vi "TSCANfd_Table.vi"(10 "y":T1(array[cluster]), 11 "MCListbox引用句柄":refnum<vi>) -> ()   [LabVIEW 2019]
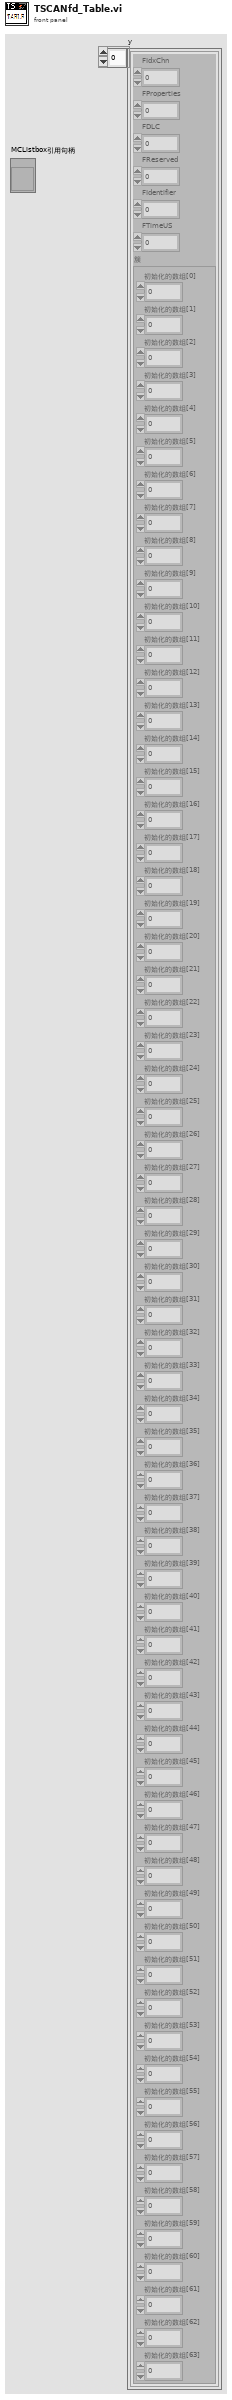
[diagram p1: front panel]
types:
  T1 = cluster{"FIdxChn":u8, "FProperties":u8, "FDLC":u8, "FReserved":u8, "FIdentifier":i32, "FTimeUS":u64, "簇":cluster{"初始化的数组[0]":u8, "初始化的数组[1]":u8, "初始化的数组[2]":u8, "初始化的数组[3]":u8, "初始化的数组[4]":u8, "初始化的数组[5]":u8, "初始化的数组[6]":u8, "初始化的数组[7]":u8, "初始化的数组[8]":u8, "初始化的数组[9]":u8, "初始化的数组[10]":u8, "初始化的数组[11]":u8, "初始化的数组[12]":u8, "初始化的数组[13]":u8, "初始化的数组[14]":u8, "初始化的数组[15]":u8, "初始化的数组[16]":u8, "初始化的数组[17]":u8, "初始化的数组[18]":u8, "初始化的数组[19]":u8, "初始化的数组[20]":u8, "初始化的数组[21]":u8, "初始化的数组[22]":u8, "初始化的数组[23]":u8, "初始化的数组[24]":u8, "初始化的数组[25]":u8, "初始化的数组[26]":u8, "初始化的数组[27]":u8, "初始化的数组[28]":u8, "初始化的数组[29]":u8, "初始化的数组[30]":u8, "初始化的数组[31]":u8, "初始化的数组[32]":u8, "初始化的数组[33]":u8, "初始化的数组[34]":u8, "初始化的数组[35]":u8, "初始化的数组[36]":u8, "初始化的数组[37]":u8, "初始化的数组[38]":u8, "初始化的数组[39]":u8, "初始化的数组[40]":u8, "初始化的数组[41]":u8, "初始化的数组[42]":u8, "初始化的数组[43]":u8, "初始化的数组[44]":u8, "初始化的数组[45]":u8, "初始化的数组[46]":u8, "初始化的数组[47]":u8, "初始化的数组[48]":u8, "初始化的数组[49]":u8, "初始化的数组[50]":u8, "初始化的数组[51]":u8, "初始化的数组[52]":u8, "初始化的数组[53]":u8, "初始化的数组[54]":u8, "初始化的数组[55]":u8, "初始化的数组[56]":u8, "初始化的数组[57]":u8, "初始化的数组[58]":u8, "初始化的数组[59]":u8, "初始化的数组[60]":u8, "初始化的数组[61]":u8, "初始化的数组[62]":u8, "初始化的数组[63]":u8}}[]
  T2 = cluster{"初始化的数组[0]":u8, "初始化的数组[1]":u8, "初始化的数组[2]":u8, "初始化的数组[3]":u8, "初始化的数组[4]":u8, "初始化的数组[5]":u8, "初始化的数组[6]":u8, "初始化的数组[7]":u8, "初始化的数组[8]":u8, "初始化的数组[9]":u8, "初始化的数组[10]":u8, "初始化的数组[11]":u8, "初始化的数组[12]":u8, "初始化的数组[13]":u8, "初始化的数组[14]":u8, "初始化的数组[15]":u8, "初始化的数组[16]":u8, "初始化的数组[17]":u8, "初始化的数组[18]":u8, "初始化的数组[19]":u8, "初始化的数组[20]":u8, "初始化的数组[21]":u8, "初始化的数组[22]":u8, "初始化的数组[23]":u8, "初始化的数组[24]":u8, "初始化的数组[25]":u8, "初始化的数组[26]":u8, "初始化的数组[27]":u8, "初始化的数组[28]":u8, "初始化的数组[29]":u8, "初始化的数组[30]":u8, "初始化的数组[31]":u8, "初始化的数组[32]":u8, "初始化的数组[33]":u8, "初始化的数组[34]":u8, "初始化的数组[35]":u8, "初始化的数组[36]":u8, "初始化的数组[37]":u8, "初始化的数组[38]":u8, "初始化的数组[39]":u8, "初始化的数组[40]":u8, "初始化的数组[41]":u8, "初始化的数组[42]":u8, "初始化的数组[43]":u8, "初始化的数组[44]":u8, "初始化的数组[45]":u8, "初始化的数组[46]":u8, "初始化的数组[47]":u8, "初始化的数组[48]":u8, "初始化的数组[49]":u8, "初始化的数组[50]":u8, "初始化的数组[51]":u8, "初始化的数组[52]":u8, "初始化的数组[53]":u8, "初始化的数组[54]":u8, "初始化的数组[55]":u8, "初始化的数组[56]":u8, "初始化的数组[57]":u8, "初始化的数组[58]":u8, "初始化的数组[59]":u8, "初始化的数组[60]":u8, "初始化的数组[61]":u8, "初始化的数组[62]":u8, "初始化的数组[63]":u8}
  T3 = typedef "LVRowAndColumnUnsignedTypeDef.ctl" = cluster{"Row":u32, "Column":u32}
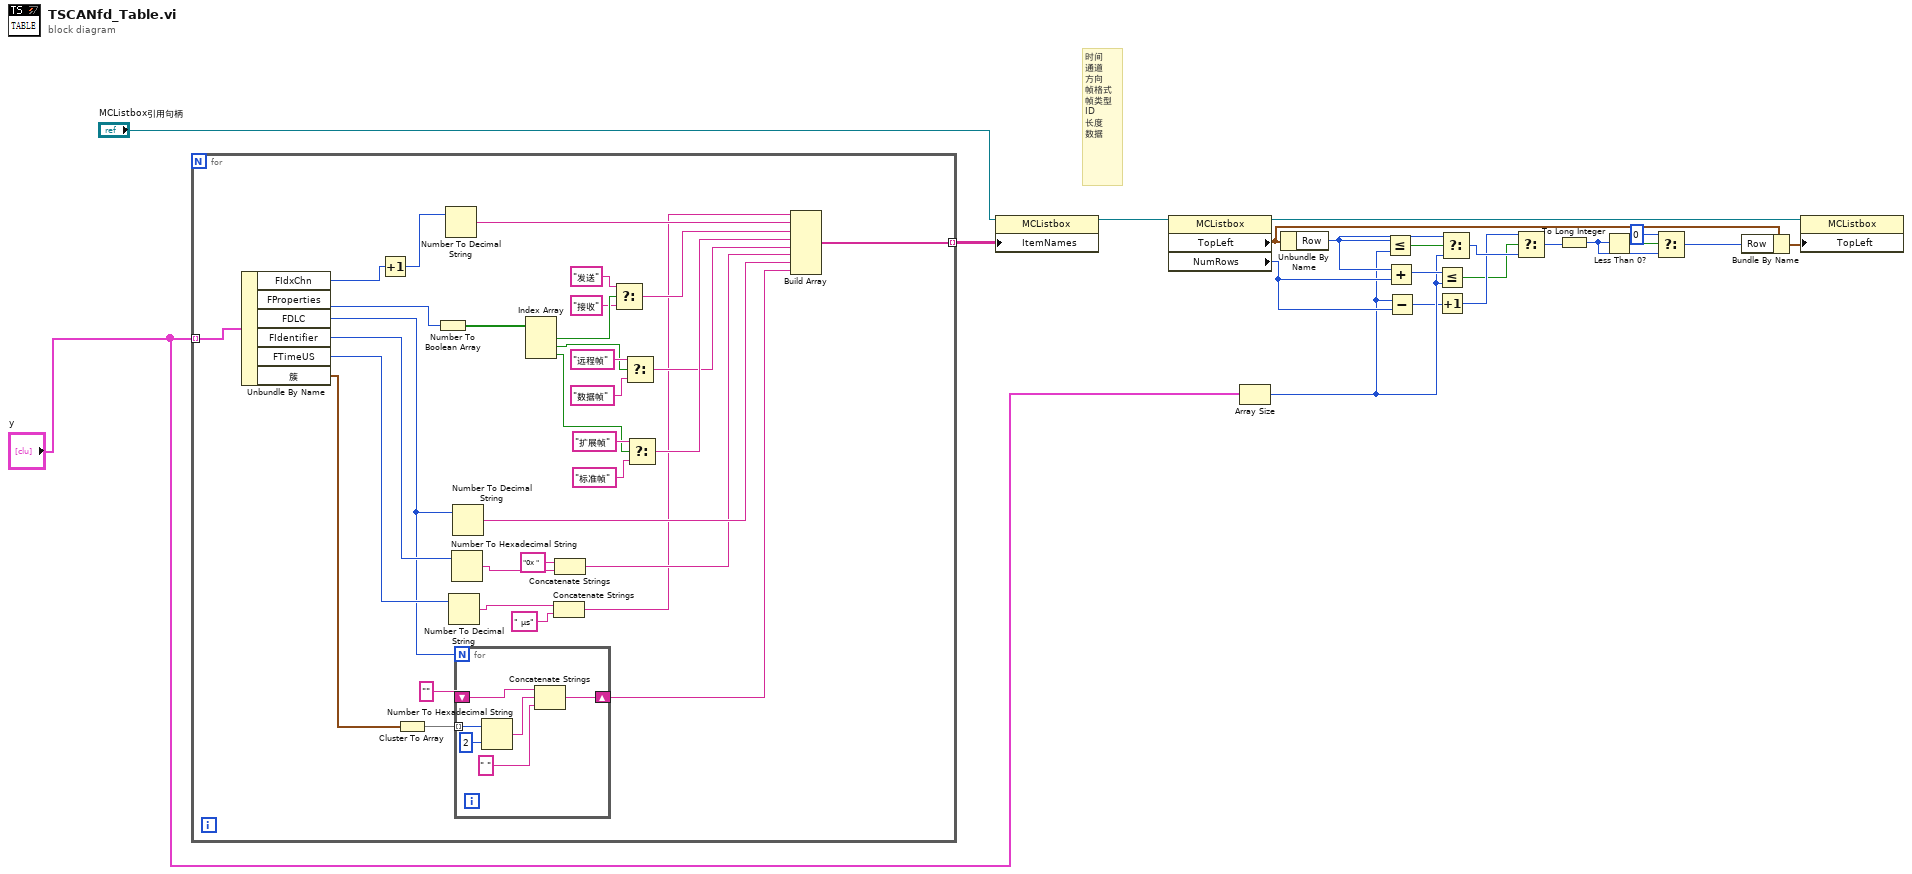
[diagram p0: block diagram]
diagram:
  # "时间\n通道\n方向\n帧格式\n帧类型\nID\n长度\n数据"
  n1 = for {
    tunnel: "y" -> [w54] mode=indexing
    tunnel: [w30] -> w21 mode=indexing
    n2 = Unbundle By Name(w54) -> ("FIdxChn"=w29:u8, "FProperties"=w53:u8, "FDLC"=w38:u8, "FIdentifier"=w42:i32, "FTimeUS"=w41:u64, "簇"=w39:T2)
    n3 = Increment(x=w29) -> (x+1=w28:u8)
    n4 = Cluster To Array(cluster=w39) -> (array=w37:u8[])
    n5 = Number To Boolean Array(number=w53) -> (Boolean array=w52:bool[])
    n6 = Number To Decimal String(number=w28) -> (decimal integer string=w36:string)  [unwired: 1 in]
    n7 = Number To Decimal String(number=w41) -> (decimal integer string=w23:string)  [unwired: 1 in]
    n8 = Number To Hexadecimal String(2:w42) -> (0:w26:string)  [unwired: 1 in]
    n9 = Number To Decimal String(number=w38) -> (decimal integer string=w32:string)  [unwired: 1 in]
    n10 = for {
      N: w38 -> [_]
      tunnel: w37 -> [w57] mode=indexing
      shift-right: [w59] -> w31
      shift-left: "" -> [w60]
      n11 = Number To Hexadecimal String(1:i16 2 ("width (-)"), 2:w57) -> (0:w56:string)
      n12 = Concatenate Strings(w60, w56, " " ("string")) -> (w59:string)
    }
    n13 = Index Array(array=w52) -> (element #1=w51:bool, element #2=w46:bool, element #3=w43:bool)  [unwired: 3 in]
    n14 = Concatenate Strings(w23, " μs" ("字符串")) -> (w24:string)
    n15 = Concatenate Strings("0x " ("字符串"), w26) -> (w27:string)
    n16 = Select(t="发送", s=w51, f="接收") -> (s? t:f=w35:string)
    n17 = Select(t="远程帧", s=w46, f="数据帧") -> (s? t:f=w33:string)
    n18 = Select(t="扩展帧", s=w43, f="标准帧") -> (s? t:f=w34:string)
    n19 = Build Array(w24, w36, w35, w34, w33, w27, w32, w31) -> (w30:string[])
  }
  n20 = property class="MCListbox"(reference="MCListbox引用句柄", "ItemNames"=w21) -> (reference out=w2:refnum<vi>)  [unwired: 1 in, 1 out]
  n21 = property class="MCListbox"(reference=w2) -> (reference out=w10:refnum<vi>, "TopLeft"=w9:T3, "NumRows"=w17:u32)  [unwired: 1 in, 1 out]
  n22 = Array Size(array="y") -> (size(s)=w15:i32)
  n23 = Unbundle By Name(w9) -> ("Row"=w18:u32)
  n24 = Less Or Equal?(x=w18, y=w15) -> (x <= y?=w19:bool)
  n25 = Add(x=w18, y=w17) -> (x+y=w16:u32)
  n26 = Subtract(x=w15, y=w17) -> (x-y=w14:u32)
  n27 = Less Or Equal?(x=w16, y=w15) -> (x <= y?=w11:bool)
  n28 = Increment(x=w14) -> (x+1=w12:u32)
  n29 = Select(t=w18, s=w19, f=w15) -> (s? t:f=w13:u32)
  n30 = Select(t=w12, s=w11, f=w13) -> (s? t:f=w8:u32)
  n31 = To Long Integer(number=w8) -> (32bit integer=w6:i32)
  n32 = Less Than 0?(x=w6) -> (x < 0?=w7:bool)
  n33 = Select(t=0, s=w7, f=w6) -> (s? t:f=w5:i32)
  n34 = Bundle By Name(cluster=w9, "Row"=w5) -> (w3:T3)
  n35 = property class="MCListbox"(reference=w10, "TopLeft"=w3) -> ()  [unwired: 1 in, 2 out]
